vi "TESTE_ENET_LNA.vi"() -> ()   [LabVIEW 2018]
uses:
  Global_Telescopio.vi
panel:
  in  "ENGENHARIA":bool
  out "element":refnum<visa-resource-name>
  out "String Enviado":string
  in  "Opcional":string
  in  "Parametro":string
  in  "Comando":u16(ring) items=["STATUS", "GIRAR", "PARAR", "MOVER"]
  in  "Dispositivo":u16(ring) items=["INDEXER", "INVERSOR", "ENCODER", "VARTRACK", "CONTROLADOR", "DOMO"]
  in  "Controlador":u16(ring) items=["RA", "DEC", "TUBO", "CUP"]
  in  "Num de Bytes a Ser lido 3":u32=10
  out "Resposta ENET 3":string
  in  "READ 3":bool
  in  "WRITE 3":bool
  # "Os Devices ENET Devem Estar Instalados e Configurados"
  # "Primeiro Aperte WRITE ENET para Enviar...\nDepois Aperte READ ENET para Ver a \nResposta..."
  # "ENET´S RS 232"
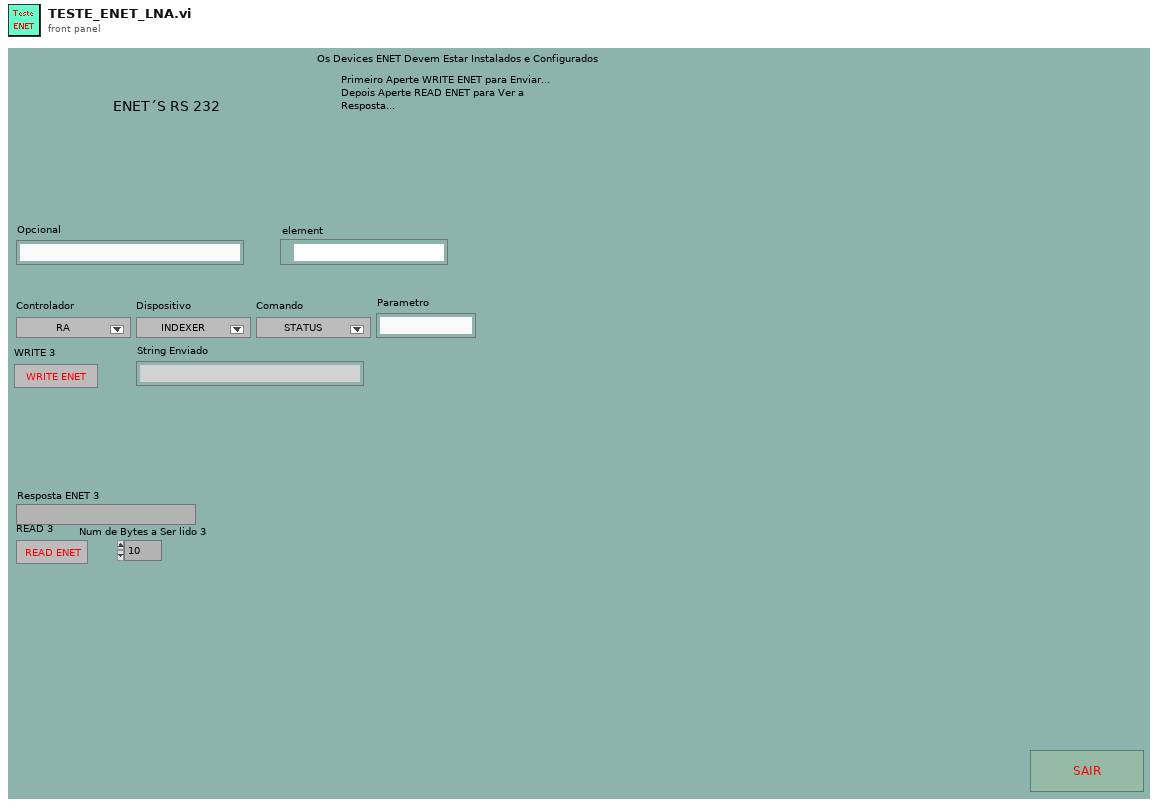
[diagram p1: front panel]
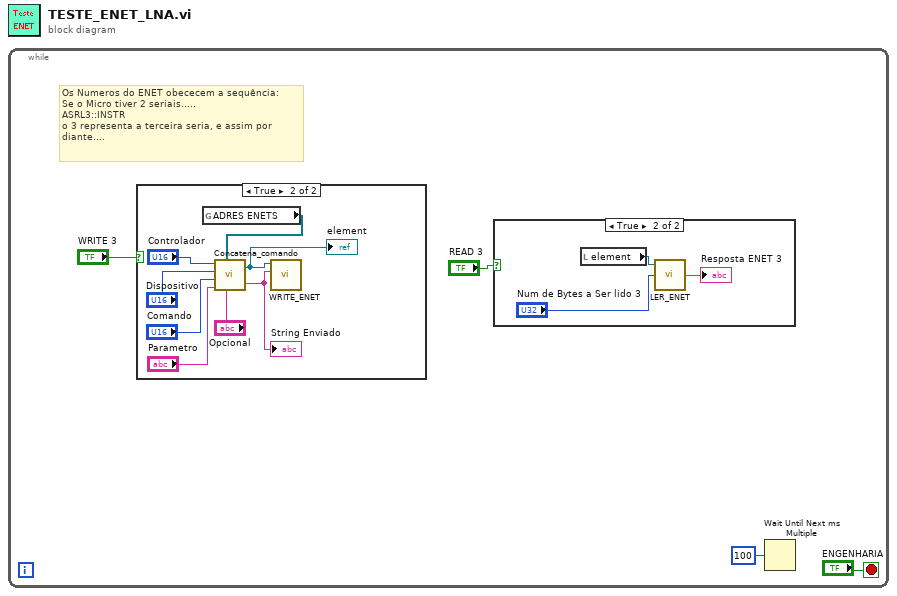
[diagram p0: block diagram]
diagram:
  n1 = while {
    stop <- "ENGENHARIA" stop-if-true
    # "Os Numeros do ENET obececem a sequência:\nSe o Micro tiver 2 seriais.....\nASRL3::INSTR\no 3 representa a terceira seria, e assim por\ndiante...."
    n2 = case shown="True" "WRITE 3" {
      frame False {
      }
      frame True {
        n3 = global read "Global_Telescopio.vi" "ADRES ENETS"() -> (w5:refnum<visa-resource-name>[])
        n4 = call "Concatena_comando.vi"("Opcional"="Opcional", "ADRES ENETS 2"=w5, "Parametro"="Parametro", "Comando"="Comando", "Dispositivo"="Dispositivo", "Controlador"="Controlador") -> ("String"=w7:string, "element"=w6:refnum<visa-resource-name>)
        "String Enviado" <- w7
        "element" <- w6
        n5 = call "WRITE_ENET.vi"("String a ser Enviado"=w7, "LNA VISA session (for class)"=w6) -> ()  [unwired: 3 in, 3 out]
      }
    }
    n6 = case shown="True" "READ 3" {
      frame False {
      }
      frame True {
        n7 = local read "element"() -> (w13:refnum<visa-resource-name>)
        n8 = call "LER_ENET.vi"("Num de Bytes a Ser lido"="Num de Bytes a Ser lido 3", "LNA VISA resource name"=w13) -> ("String Lida"=→"Resposta ENET 3":string)  [unwired: 1 in, 2 out]
      }
    }
    n9 = Wait Until Next ms Multiple(millisecond multiple=u32 100) -> ()  [unwired: 1 out]
  }
